vi "Stream LLP Packets to Disk.vi"(0 "fpga interface in":refnum<k20>, 1 "bytes acquired indicator ref":refnum<vi>, 5 "serial input channel":string, 7 "base packet file path":path, 9 "fetch size (elements)":u32=40960, 11 "error in (no error)":errorcluster, 12 "fetch timeout (s)":dbl=1.0, 13 "log to disk":bool=TRUE) -> (4 "fpga interface out":refnum<k20>, 6 "file path out":path, 8 "acquisition error":bool, 15 "error out":errorcluster)   [LabVIEW 2025, in "GettingStarted_Acq_148X_Host.lvlib"]
uses:
  GettingStarted_Acq_148X_Host.lvlib
  <vilib>/rvi/interface/nirviMethod/nirviMethod.xnode
  <vilib>/rvi/interface/nirviReadWriteControl/nirviReadWriteControl.xnode
  <vilib>/FPGAPlugInAG/Dynamic/niLvFpga_AcquireReadRegionFifo_Dynamic.vi
  <vilib>/rvi/errors/niLvFpgaMergeErrorWithErrorCode.vi
  <instrlib>/FlexRIO/Automotive Vision Utility/v1/Host/Automotive Vision Utility.lvlib
  Types/148x_Acq_FPGA_Reference.ctl
  0829f115-c11d-4785-86b3-38f743f517d6.vi
  Common/GettingStarted_Common_148X_Host.lvlib
  NiFpgaLv.dll
  <vilib>/rvi/interface/Simulation/niFpgaSimulationCallBeginRW.vi
  <vilib>/rvi/errors/niLvFpgaAdjustHostInterfaceError.vi
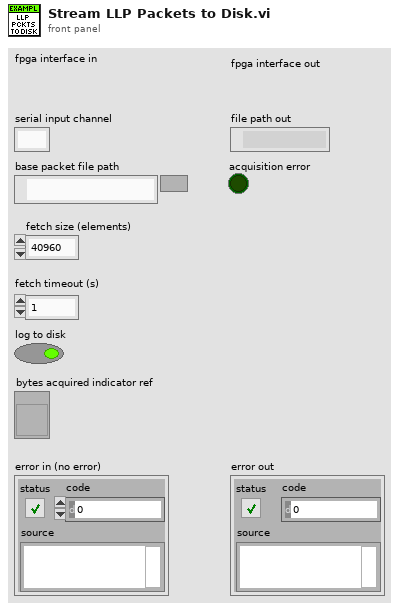
[diagram p1: front panel]
types:
  T1 = typedef "Automotive Vision Utility.lvlib/Serial Channel Type.ctl" = enum16{"Serial Input Channel", "Serial Output Channel", "Unknown Channel Type"}
  T2 = typedef "GettingStarted_Acq_148X_Host.lvlib/148x_Acq_FPGA_Reference.ctl" = refnum<k20>
  T3 = enum16{"open", "open or create", "create or replace", "create", "open (read-only)"}
  T4 = cluster{"acq state":enum8{"Idle", "Wait for First Packet Header", "Acquire", "Wait for Last Packet Header", "Wait for End of Last Packet"}, "stop timed out":bool, "bad packet header":bool, "bad packet payload":bool, "bad packet size":bool, "dram status":cluster{"bytes written":u64, "bytes read":u64, "overflow":bool, "partition full":bool, "last byte flushed":bool}}[]
  T5 = cluster{"acq state":enum8{"Idle", "Wait for First Packet Header", "Acquire", "Wait for Last Packet Header", "Wait for End of Last Packet"}, "stop timed out":bool, "bad packet header":bool, "bad packet payload":bool, "bad packet size":bool, "dram status":cluster{"bytes written":u64, "bytes read":u64, "overflow":bool, "partition full":bool, "last byte flushed":bool}}
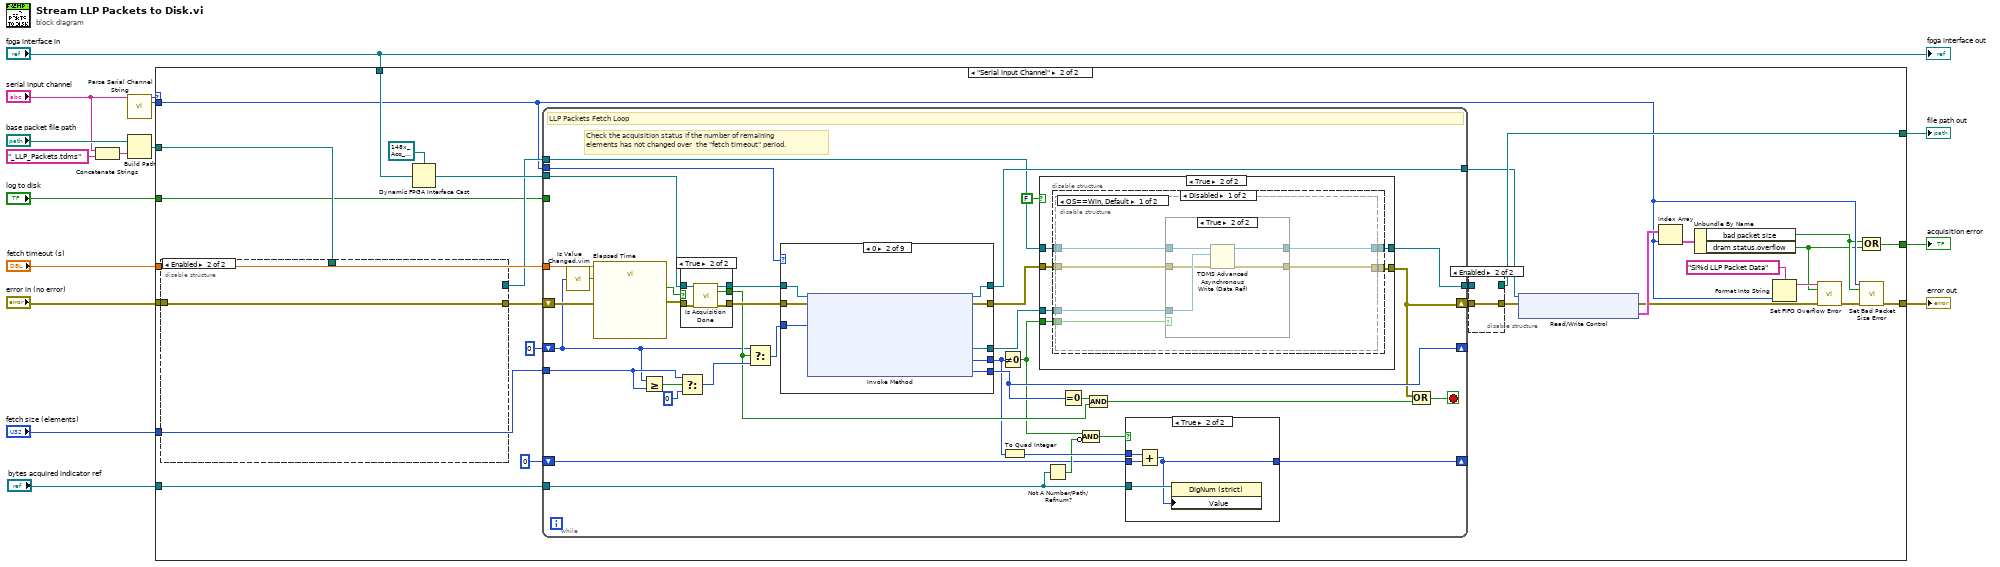
[diagram p0: block diagram]
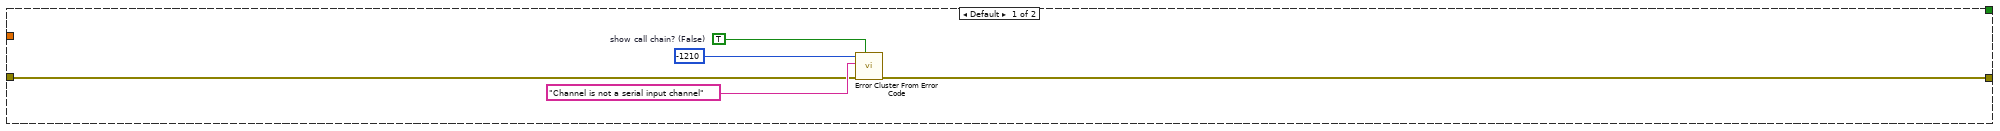
[diagram p2: hidden frame]
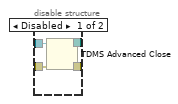
[diagram p3: hidden frame]
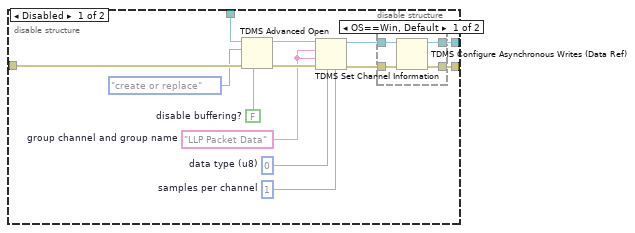
[diagram p4: hidden frame]
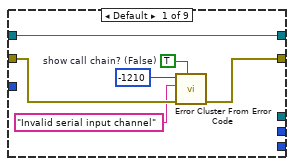
[diagram p8: hidden frame]
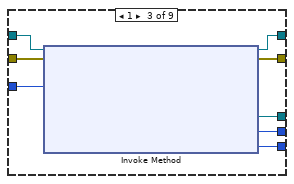
[diagram p9: hidden frame]
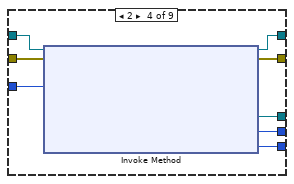
[diagram p10: hidden frame]
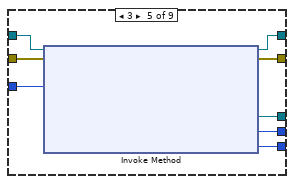
[diagram p11: hidden frame]
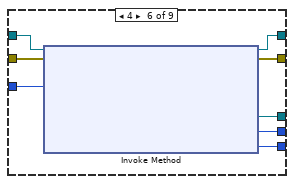
[diagram p12: hidden frame]
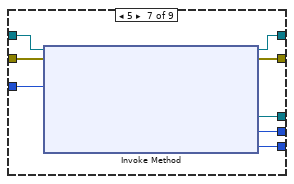
[diagram p13: hidden frame]
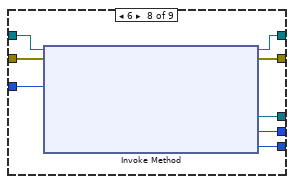
[diagram p14: hidden frame]
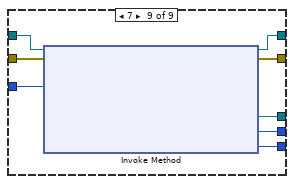
[diagram p15: hidden frame]
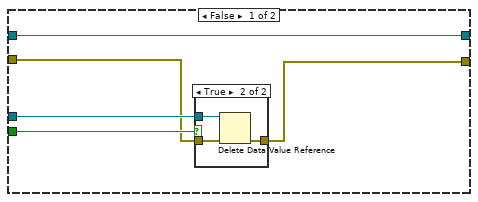
[diagram p16: hidden frame]
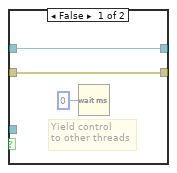
[diagram p18: hidden frame]
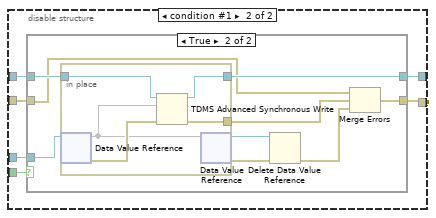
[diagram p19: hidden frame]
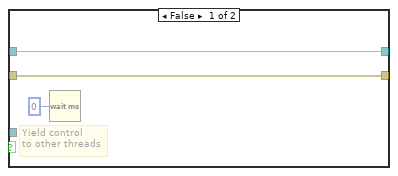
[diagram p20: hidden frame]
diagram:
  n1 = Concatenate Strings("serial input channel", "_LLP_Packets.tdms") -> (w9:string)
  n2 = call <instrlib>:"Parse Serial Channel String.vi"("serial channel string"="serial input channel") -> ("serial channel type"=w12:T1, "channel number"=w13:i32)  [unwired: 13 in]
  n3 = Build Path(base path="base packet file path", name or relative path=w9) -> (appended path=w6:path)
  n4 = case shown="\"Serial Input Channel\"" w12 {
    tunnel: "error in (no error)" -> [w18 w50]
    tunnel: w6 -> [_ w46]
    tunnel: [w17 w26] -> w15
    tunnel: [_ w22] -> w14
    tunnel: w13 -> [_ w25]
    tunnel: "fetch size (elements)" -> [_ w44]
    tunnel: "fpga interface in" -> [_ w43]
    tunnel: [_ w40] -> w5
    tunnel: "fetch timeout (s)" -> [_ w39]
    tunnel: "log to disk" -> [_ w30]
    tunnel: "bytes acquired indicator ref" -> [_ w28]
    frame Default {
      w19 = TRUE  # show call chain? (False)
      n5 = call <vilib>:"Error Cluster From Error Code.vi"("show call chain? (False)"=w19, "error in (no error)"=w18, "error message (\"\")"="Channel is not a serial input channel" ("error message (\"\")"), "error code (0)"=-1210) -> ("error out"=w17:errorcluster)  [unwired: 5 in]
    }
    frame "Serial Input Channel" {
      n6 = disable-structure shown="Enabled" {
        disable-tunnel: w50 -> [w68 w75]
        disable-tunnel: w46 -> [w65 _]
        disable-tunnel: [w58 _] -> w35
        disable-tunnel: [w57 w75] -> w34
        frame Disabled {
          w66 = u32 1  # samples per channel
          w63 = FALSE  # disable buffering?
          w62 = u8 0  # data type (u8)
          w60 = "LLP Packet Data"  # group channel and group name
          n7 = TDMS Advanced Open(6:w63, 8:w68, 10:T3."create or replace" ("operation (0:open)"), 11:w65) -> (0:w61:errorcluster, 3:w67:refnum<k34>)  [unwired: 1 in, 1 out]
          n8 = TDMS Set Channel Information(4:w66, 6:w62, 8:w61, 9:w60, 10:w60, 11:w67) -> (0:w56:errorcluster, 3:w59:refnum<k34>)  [unwired: 1 in]
          n9 = disable-structure shown="OS==Win, Default" {
            disable-tunnel: w56 -> [w69 w74]
            disable-tunnel: [w72 w73] -> w58
            disable-tunnel: [w71 w74] -> w57
            disable-tunnel: w59 -> [w70 w73]
            frame condition #0 (active) {
              n10 = TDMS Configure Asynchronous Writes (Data Ref)(8:w69, 11:w70) -> (0:w71:errorcluster, 3:w72:refnum<k34>)  [unwired: 2 in]
            }
            frame condition #1 {
            }
          }
        }
        frame Enabled {
        }
      }
      n11 = Dynamic FPGA Interface Cast(Session In=T2 refnum ("FPGA VI Reference Out"), Type=w43) -> (Session Out=w41:T2)
      n12 = while {
        shift-right: [w88] -> w49
        shift-left: w34 -> [w94]
        tunnel: w41 -> [w98]
        shift-right: [w90] -> _
        shift-left: u32 0 ("Elements Remaining") -> [w91]
        tunnel: w35 -> [w87]
        tunnel: [w89] -> w47
        tunnel: [w106] -> w37
        tunnel: w25 -> [w109]
        tunnel: w44 -> [w100]
        tunnel: w39 -> [w105]
        tunnel: w30 -> [_]
        shift-right: [w79] -> _
        shift-left: i64 0 -> [w78]
        tunnel: w28 -> [w80]
        stop <- w110 stop-if-true
        # "Check the acquisition status if the number of remaining \nelements has not changed over  the \"fetch timeout\" period."
        # "LLP Packets Fetch Loop"
        n13 = call "Is Value Changed.vim"("value"=w91) -> ("changed or first call?"=w104:bool)
        n14 = call "Elapsed Time"("Time Target (s)"=w105, "Reset"=w104, "error in (no error)"=w94) -> ("Time has Elapsed"=w96:bool, "error out"=w93:errorcluster)  [unwired: 9 in, 6 out]
        n15 = Greater Or Equal?(x=w91, y=w100) -> (x >= y?=w103:bool)
        n16 = case shown="True" w96 {
          tunnel: w93 -> [w117 w122]
          tunnel: [w117 w121] -> w99
          tunnel: w98 -> [w116 w120]
          tunnel: [w116 w119] -> w97
          tunnel: [_ w118] -> w95
          frame False {
          }
          frame True {
            n17 = call "Is Acquisition Done.vi"("fpga interface in"=w120, "error in (no error)"=w122) -> ("fpga interface out"=w119:T2, "acquisition done"=w118:bool, "error out"=w121:errorcluster)  [unwired: 11 in]
          }
        }
        n18 = Select(t=w100, s=w103, f=u32 0 ("Elements Remaining")) -> (s? t:f=w101:u32)
        n19 = Select(t=w91, s=w95, f=w101) -> (s? t:f=w102:u32)
        n20 = case shown="0" w109 {
          tunnel: w97 -> [w128 w136 w144 w152 w160 w168 w176 w184 w192]
          tunnel: w99 -> [w127 w135 w143 w151 w159 w167 w175 w183 w191]
          tunnel: [_ w134 w142 w150 w158 w166 w174 w182 w190] -> w85
          tunnel: [_ w133 w141 w149 w157 w165 w173 w181 w189] -> w77
          tunnel: w102 -> [_ w132 w140 w148 w156 w164 w172 w180 w188]
          tunnel: [w124 w130 w138 w146 w154 w162 w170 w178 w186] -> w86
          tunnel: [_ w131 w139 w147 w155 w163 w171 w179 w187] -> w90
          tunnel: [w128 w129 w137 w145 w153 w161 w169 w177 w185] -> w106
          frame Default {
            w123 = TRUE  # show call chain? (False)
            n21 = call <vilib>:"Error Cluster From Error Code.vi"("show call chain? (False)"=w123, "error in (no error)"=w127, "error message (\"\")"="Invalid serial input channel" ("error message (\"\")"), "error code (0)"=-1210) -> ("error out"=w124:errorcluster)  [unwired: 5 in]
          }
          frame 0 {
            n22 = xnode "Invoke Method"("FPGA VI Reference In"=w136, "error in"=w135, "Number of Elements"=w132) -> ("FPGA VI Reference Out"=w129:T2, "error out"=w130:errorcluster, "Read Region Reference"=w134:refnum<data-value>, "Elements In Region"=w133:u32, "Elements Remaining"=w131:u32)  [unwired: 1 in]
          }
          frame 1 {
            n23 = xnode "Invoke Method"("FPGA VI Reference In"=w144, "error in"=w143, "Number of Elements"=w140) -> ("FPGA VI Reference Out"=w137:T2, "error out"=w138:errorcluster, "Read Region Reference"=w142:refnum<data-value>, "Elements In Region"=w141:u32, "Elements Remaining"=w139:u32)  [unwired: 1 in]
          }
          frame 2 {
            n24 = xnode "Invoke Method"("FPGA VI Reference In"=w152, "error in"=w151, "Number of Elements"=w148) -> ("FPGA VI Reference Out"=w145:T2, "error out"=w146:errorcluster, "Read Region Reference"=w150:refnum<data-value>, "Elements In Region"=w149:u32, "Elements Remaining"=w147:u32)  [unwired: 1 in]
          }
          frame 3 {
            n25 = xnode "Invoke Method"("FPGA VI Reference In"=w160, "error in"=w159, "Number of Elements"=w156) -> ("FPGA VI Reference Out"=w153:T2, "error out"=w154:errorcluster, "Read Region Reference"=w158:refnum<data-value>, "Elements In Region"=w157:u32, "Elements Remaining"=w155:u32)  [unwired: 1 in]
          }
          frame 4 {
            n26 = xnode "Invoke Method"("FPGA VI Reference In"=w168, "error in"=w167, "Number of Elements"=w164) -> ("FPGA VI Reference Out"=w161:T2, "error out"=w162:errorcluster, "Read Region Reference"=w166:refnum<data-value>, "Elements In Region"=w165:u32, "Elements Remaining"=w163:u32)  [unwired: 1 in]
          }
          frame 5 {
            n27 = xnode "Invoke Method"("FPGA VI Reference In"=w176, "error in"=w175, "Number of Elements"=w172) -> ("FPGA VI Reference Out"=w169:T2, "error out"=w170:errorcluster, "Read Region Reference"=w174:refnum<data-value>, "Elements In Region"=w173:u32, "Elements Remaining"=w171:u32)  [unwired: 1 in]
          }
          frame 6 {
            n28 = xnode "Invoke Method"("FPGA VI Reference In"=w184, "error in"=w183, "Number of Elements"=w180) -> ("FPGA VI Reference Out"=w177:T2, "error out"=w178:errorcluster, "Read Region Reference"=w182:refnum<data-value>, "Elements In Region"=w181:u32, "Elements Remaining"=w179:u32)  [unwired: 1 in]
          }
          frame 7 {
            n29 = xnode "Invoke Method"("FPGA VI Reference In"=w192, "error in"=w191, "Number of Elements"=w188) -> ("FPGA VI Reference Out"=w185:T2, "error out"=w186:errorcluster, "Read Region Reference"=w190:refnum<data-value>, "Elements In Region"=w189:u32, "Elements Remaining"=w187:u32)  [unwired: 1 in]
          }
        }
        n30 = Not Equal To 0?(x=w77) -> (x != 0?=w81:bool)
        n31 = To Quad Integer(1:w77) -> (0:w84:i64)
        n32 = case shown="True" FALSE {
          tunnel: w87 -> [w197 w207]
          tunnel: w86 -> [w194 w206]
          tunnel: w85 -> [w196 w205]
          tunnel: [w197 w204] -> w89
          tunnel: [w193 w203] -> w88
          tunnel: w81 -> [w195 w202]
          frame False {
            n33 = case shown="True" w195 {
              tunnel: w194 -> [w198 w201]
              tunnel: w196 -> [_ w200]
              tunnel: [w198 w199] -> w193
              frame False {
              }
              frame True {
                n34 = Delete Data Value Reference(data value reference=w200, error in=w201) -> (error out=w199:errorcluster)  [unwired: 1 out]
              }
            }
          }
          frame True {
            n35 = disable-structure shown="Disabled" {
              disable-tunnel: w207 -> [w213 w252]
              disable-tunnel: w206 -> [w212 w251]
              disable-tunnel: w205 -> [w211 _]
              disable-tunnel: [w210 w252] -> w204
              disable-tunnel: [w209 w251] -> w203
              disable-tunnel: w202 -> [w208 _]
              frame Disabled {
                n36 = disable-structure shown="OS==Win, Default" {
                  disable-tunnel: w213 -> [w217 w233]
                  disable-tunnel: w212 -> [w216 w232]
                  disable-tunnel: w211 -> [w215 w231]
                  disable-tunnel: w208 -> [w214 w230]
                  disable-tunnel: [w219 w229] -> w210
                  disable-tunnel: [w218 w228] -> w209
                  frame condition #0 (active) {
                    n37 = case shown="True" w214 {
                      tunnel: w217 -> [w221 w227]
                      tunnel: [w221 w225] -> w219
                      tunnel: w216 -> [w220 w223]
                      tunnel: [w220 w224] -> w218
                      tunnel: w215 -> [_ w226]
                      frame False {
                        # "Yield control\nto other threads"
                        n38 = Wait (ms)(milliseconds to wait=u32 0) -> ()  [unwired: 1 out]
                      }
                      frame True {
                        n39 = TDMS Advanced Asynchronous Write (Data Ref)(8:w223, 10:w226, 11:w227) -> (0:w224:errorcluster, 3:w225:refnum<k34>)  [unwired: 1 in]
                      }
                    }
                  }
                  frame condition #1 {
                    n40 = case shown="True" w230 {
                      tunnel: w233 -> [w235 w244]
                      tunnel: [w235 w241] -> w229
                      tunnel: w232 -> [w234 w240]
                      tunnel: [w234 w237] -> w228
                      tunnel: w231 -> [_ w245]
                      frame False {
                        # "Yield control\nto other threads"
                        n41 = Wait (ms)(milliseconds to wait=u32 0) -> ()  [unwired: 1 out]
                      }
                      frame True {
                        n42 = in-place {
                          in-place-border: w244 -> [w250]
                          in-place-border: [w247] -> w239
                          in-place-border: [w246] -> w241
                          n43 = in-place-dvr #1(w245) -> (w248:u8[], w249:errorcluster)
                          n44 = TDMS Advanced Synchronous Write(8:w249, 10:w248, 11:w250) -> (0:w247:errorcluster, 3:w246:refnum<k34>)
                          n45 = in-place-dvr #1(w248) -> (w242:refnum<data-value>, w243:errorcluster)
                        }
                        n46 = Delete Data Value Reference(data value reference=w242, error in=w243) -> (error out=w238:errorcluster)  [unwired: 1 out]
                        n47 = Merge Errors(w240, w239, w238) -> (w237:errorcluster)
                      }
                    }
                  }
                }
              }
              frame Enabled {
              }
            }
          }
        }
        n48 = Not A Number/Path/Refnum?(number/path/refnum=w80) -> (NaN/Path/Refnum?=w82:bool)
        n49 = Equal To 0?(x=w90) -> (x = 0?=w92:bool)
        n50 = Compound Arithmetic op=AND(w81, invert w82) -> (w83:bool)
        n51 = Compound Arithmetic op=AND(w92, w95) -> (w107:bool)
        n52 = case shown="True" w83 {
          tunnel: w78 -> [w111 w115]
          tunnel: w84 -> [_ w114]
          tunnel: [w111 w112] -> w79
          tunnel: w80 -> [_ w113]
          frame False {
          }
          frame True {
            n53 = Add(x=w114, y=w115) -> (x+y=w112:i64)
            n54 = property class="DigNum (strict)"(reference=w113, "Value"=w112) -> ()  [unwired: 1 in, 2 out]
          }
        }
        n55 = Compound Arithmetic op=OR(w88, w107) -> (w110:bool)
      }
      n56 = disable-structure shown="Enabled" {
        disable-tunnel: w49 -> [w54 w55]
        disable-tunnel: w47 -> [w53 _]
        disable-tunnel: [w52 _] -> w40
        disable-tunnel: [w51 w55] -> w38
        frame Disabled {
          n57 = TDMS Advanced Close(8:w54, 11:w53) -> (0:w51:errorcluster, 3:w52:path)  [unwired: 2 in]
        }
        frame Enabled {
        }
      }
      n58 = xnode "Read/Write Control"("FPGA VI Reference In"=w37, "error in"=w38) -> ("error out"=w33:errorcluster, "serial input channel status"=w36:T4)  [unwired: 1 out]
      n59 = Index Array(array=w36, index=w25) -> (element=w45:T5)
      n60 = Unbundle By Name(w45) -> ("bad packet size"=w24:bool, "dram status.overflow"=w23:bool)
      n61 = Format Into String(format string="SI%d LLP Packet Data" ("fifo name"), w25) -> (resulting string=w32:string)  [unwired: 2 in, 1 out]
      n62 = call "Set FIFO Overflow Error.vi"("fifo name"=w32, "overflow"=w23, "error in (no error)"=w33) -> ("error out"=w27:errorcluster)  [unwired: 12 in]
      n63 = call "Set Bad Packet Size Error.vi"("serial input channel"=w25, "bad packet size"=w24, "error in (no error)"=w27) -> ("error out"=w26:errorcluster)  [unwired: 12 in]
      n64 = Compound Arithmetic op=OR(w24, w23) -> (w22:bool)
    }
  }
  "error out" <- w15
  "acquisition error" <- w14
  "file path out" <- w5
  "fpga interface out" <- "fpga interface in"
